vi "ImpulsatorC.vi"(7 "Initialise":bool, 10 "PV":dbl format="%#.1g", 11 "Impulsator in":refnum<class "Impulsator.lvclass">) -> (2 "YB":bool, 3 "Impulsator out":refnum<class "Impulsator.lvclass">)   [LabVIEW 2019, in "Userlib.lvlib" / "Impulsator.lvclass"]
uses:
  Impulsator.lvclass
  Impulsator.lvclass/Impulsator.ctl
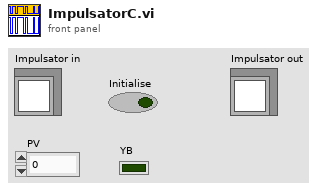
[diagram p1: front panel]
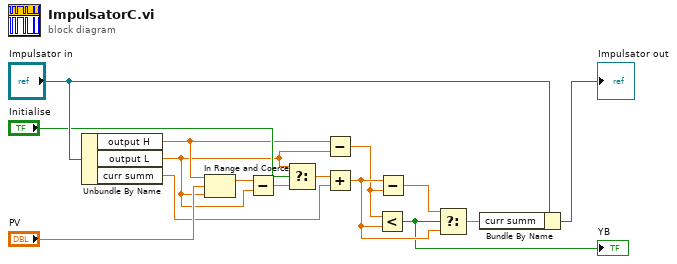
[diagram p0: block diagram]
diagram:
  n1 = Unbundle By Name("Impulsator in") -> ("output H"=w3:dbl, "output L"=w1:dbl, "curr summ"=w4:dbl)
  n2 = In Range and Coerce(upper limit=w3, x="PV", lower limit=w1) -> (coerced(x)=w6:dbl)  [unwired: 1 out]
  n3 = Subtract(x=w6, y=w1) -> (x-y=w5:dbl)
  n4 = Select(t=w1, s="Initialise", f=w5) -> (s? t:f=w13:dbl)
  n5 = Subtract(x=w3, y=w1) -> (x-y=w2:dbl)
  n6 = Add(x=w13, y=w4) -> (x+y=w10:dbl)
  n7 = Less?(x=w2, y=w10) -> (x < y?=w9:bool)
  "YB" <- w9
  n8 = Subtract(x=w10, y=w2) -> (x-y=w11:dbl)
  n9 = Select(t=w11, s=w9, f=w10) -> (s? t:f=w7:dbl)
  n10 = Bundle By Name(cluster="Impulsator in", "curr summ"=w7) -> (→"Impulsator out":refnum<class "Impulsator.lvclass">)
